vi "LtaParseArg.vi"(10 "Arg In":string="doe1.ray.mi") -> (0 "ArgRemaining":string="ray.mi", 1 "Arg 1":string="doe", 2 "Arg1Num":i32=1)   [LabVIEW 2014, in "Test.lvclass"]
uses:
  Test.lvclass
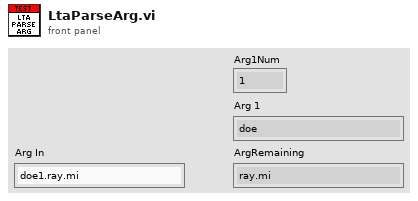
[diagram p1: front panel]
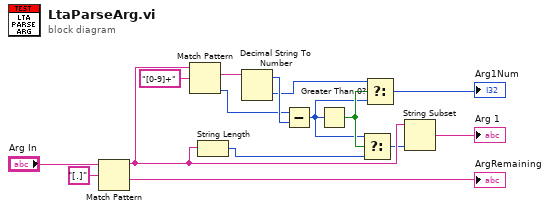
[diagram p0: block diagram]
diagram:
  n1 = Match Pattern(string="Arg In", regular expression="[.]") -> (before substring=w8:string, after substring=→"ArgRemaining":string)  [unwired: 1 in, 2 out]
  n2 = Match Pattern(string=w8, regular expression="[0-9]+") -> (match substring=w11:string, offset past match=w9:i32)  [unwired: 1 in, 2 out]
  n3 = String Length(string=w8) -> (length=w6:i32)
  n4 = Decimal String To Number(string=w11) -> (offset past number=w10:i32, number=w4:i32)  [unwired: 2 in]
  n5 = Subtract(x=w9, y=w10) -> (x-y=w3:i32)
  n6 = Greater Than 0?(x=w3) -> (x > 0?=w5:bool)
  n7 = Select(t=w3, s=w5, f=w6) -> (s? t:f=w7:i32)
  n8 = Select(t=w4, s=w5, f=w3) -> (s? t:f=→"Arg1Num":i32)
  n9 = String Subset(string=w8, length (rest)=w7) -> (substring=→"Arg 1":string)  [unwired: 1 in]
